vi "Parse CD XML.vi"(8 "error in (no error)":errorcluster, 10 "Custom Device XML Schema":path, 11 "Custom Device XML":path) -> (0 "error out":errorcluster, 3 "Custom Device Information":T1 {"Driver VIs"."Supported Target" items=["All", "Pharlap", "VxWorks", "Windows", "Linux_32_ARM", "Linux_x64", "PharlapWindows", "PharlapVxWorks", "VxWorksWindows"]; "Driver VIs"."Type" items=["Absolute", "ToBase", "ToCommonDocDir", "ToApplicationDataDir"]; "Execution Mode" items=["Asynchronous", "InlineHWInterface", "InlineModelInterface", "InlineTimingandSync", "AsynchronousTimingandSync"]})   [LabVIEW 2017, in "VeriStand SLSC Scripting.lvlib"]
uses:
  VeriStand SLSC Scripting.lvlib
  Controls/Custom Device Information.ctl
  Controls/Driver VI Information.ctl
  NationalInstruments.VeriStand.XMLReader
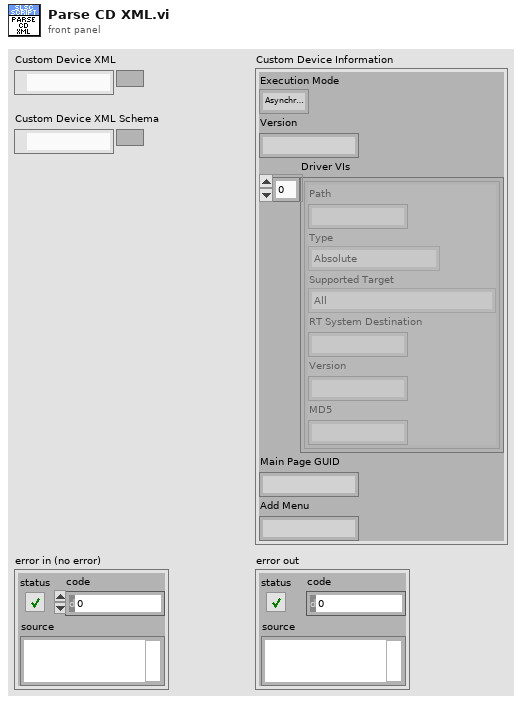
[diagram p1: front panel]
types:
  T1 = typedef "VeriStand SLSC Scripting.lvlib/Custom Device Information.ctl" = cluster{"Execution Mode":i32, "Version":string, "Driver VIs":T2[], "Main Page GUID":string, "Add Menu":string}
  T2 = typedef "VeriStand SLSC Scripting.lvlib/Driver VI Information.ctl" = cluster{"Path":string, "Type":i32, "Supported Target":i32, "RT System Destination":string, "Version":string, "MD5":string}
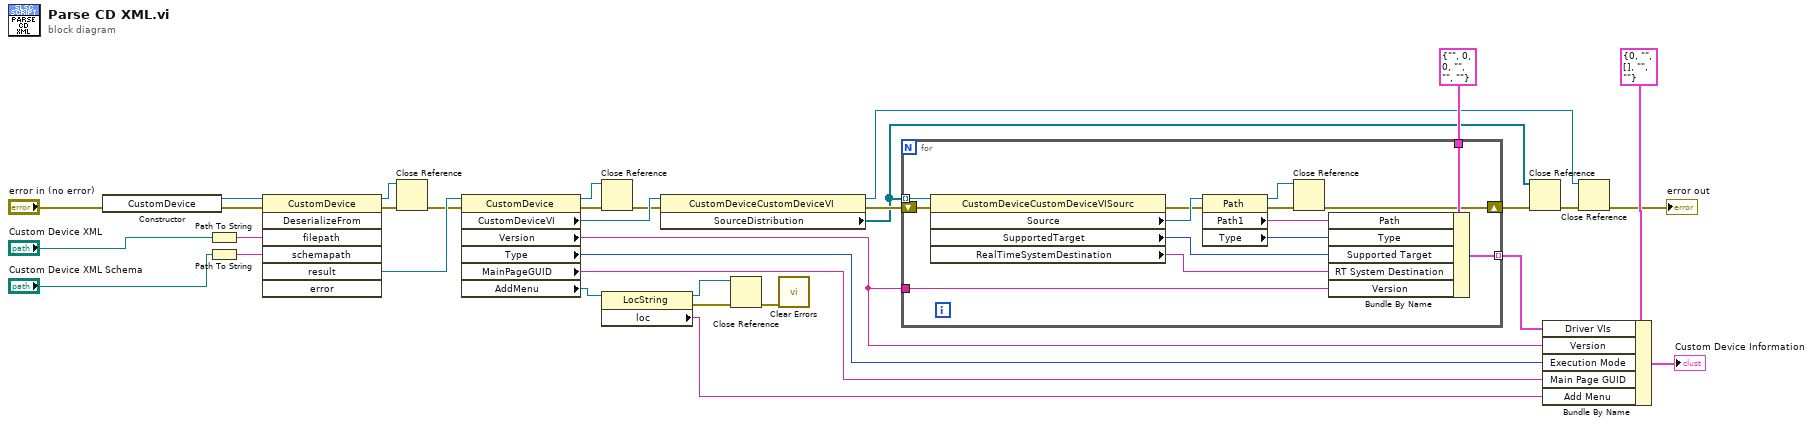
[diagram p0: block diagram]
diagram:
  n1 = constructor class="CustomDevice"(error in="error in (no error)") -> (reference out=w29:refnum<k24>, error out=w28:errorcluster)  [unwired: 2 in, 1 out]
  n2 = Path To String(path="Custom Device XML") -> (string=w32:string)
  n3 = Path To String(path="Custom Device XML Schema") -> (string=w30:string)
  n4 = invoke class="CustomDevice" method="DeserializeFrom"(reference=w29, error in=w28, "filepath"=w32, "schemapath"=w30) -> (reference out=w26:refnum<k24>, error out=w27:errorcluster, "result"=w25:refnum<k24>)  [unwired: 3 in, 4 out]
  n5 = Close Reference(reference=w26, error in (no error)=w27) -> (error out=w15:errorcluster)
  n6 = property class="CustomDevice"(reference=w25, error in=w15) -> (reference out=w7:refnum<k24>, error out=w23:errorcluster, "CustomDeviceVI"=w24:refnum<k24>, "Version"=w20:string, "Type"=w19:i32, "MainPageGUID"=w6:string, "AddMenu"=w5:refnum<k24>)
  n7 = Close Reference(reference=w7, error in (no error)=w23) -> (error out=w8:errorcluster)
  n8 = property class="LocString"(reference=w5) -> (reference out=w3:refnum<k24>, error out=w4:errorcluster, "loc"=w2:string)  [unwired: 1 in]
  n9 = property class="CustomDeviceCustomDeviceVI"(reference=w24, error in=w8) -> (reference out=w10:refnum<k24>, error out=w14:errorcluster, "SourceDistribution"=w12:refnum<k24>[])
  n10 = Close Reference(reference=w3, error in (no error)=w4) -> (error out=w1:errorcluster)
  n11 = call <vilib>:"Clear Errors.vi"("error in (no error)"=w1) -> ()  [unwired: 5 in, 2 out]
  n12 = for {
    tunnel: w12 -> [w47] mode=indexing
    tunnel: T2 {"Path"="", "Type"=0, "Supported Target"=0, "RT System Destination"="", "Version"="", "MD5"=""} ("Driver VI Information") -> [w45]
    tunnel: [w40] -> w17 mode=indexing
    tunnel: w20 -> [w39]
    shift-right: [w35] -> w13
    shift-left: w14 -> [w38]
    n13 = property class="CustomDeviceCustomDeviceVISourc"(reference=w47, error in=w38) -> (error out=w37:errorcluster, "Source"=w46:refnum<k24>, "SupportedTarget"=w42:i32, "RealTimeSystemDestination"=w41:string)  [unwired: 1 out]
    n14 = property class="Path"(reference=w46, error in=w37) -> (reference out=w34:refnum<k24>, error out=w36:errorcluster, "Path1"=w44:string, "Type"=w43:i32)
    n15 = Close Reference(reference=w34, error in (no error)=w36) -> (error out=w35:errorcluster)
    n16 = Bundle By Name(cluster=w45, "Path"=w44, "Type"=w43, "Supported Target"=w42, "RT System Destination"=w41, "Version"=w39) -> (w40:T2)
  }
  n17 = Close Reference(reference=w12, error in (no error)=w13) -> (error out=w11:errorcluster)
  n18 = Bundle By Name(cluster=T1 {"Execution Mode"=0, "Version"="", "Driver VIs"=[], "Main Page GUID"="", "Add Menu"=""} ("Custom Device Information"), "Driver VIs"=w17, "Version"=w20, "Execution Mode"=w19, "Main Page GUID"=w6, "Add Menu"=w2) -> (→"Custom Device Information":T1)
  n19 = Close Reference(reference=w10, error in (no error)=w11) -> (error out=→"error out":errorcluster)
